vi "PH_TKTDS-30xx.Reset.vi"(0 "i ref in":refnum<vi>, 5 "error IO":errorcluster) -> (14 "i ref out":refnum<vi>, 19 "error out":errorcluster)   [LabVIEW 2014, in "PH_TKTDS-30xx.lvlib"]
doc: "If the connection is established, this VO resets the hardware. It queries the errors which are written to own attributes, if the value has changed."
uses:
  PH_TKTDS-30xx.lvlib
  instr.lib/TKDS3032-PHELIX/tktds3032-PHELIX - Driver np.lvlib
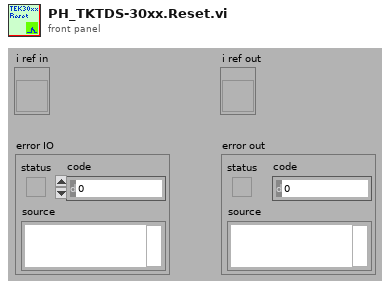
[diagram p1: front panel]
types:
  T1 = typedef "PH_TKTDS-30xx.lvlib/PH_TKTDS-30xx.i attribute.ctl" = cluster{"Default VISA Resource":string, "VISA Resource Name":refnum<visa-resource-name>, "Revision":cluster{"Instrument Driver":string, "Instrument Firmware":string}, "Selftest":cluster{"Result":u32, "Message":string}, "Channels":T2[], "Trigger Configuration":T3, "Acquisition Configuration":T4, "Fetched Waveforms":T5[], "GUI Refs":T6, "GUI Refs Channels":refnum<vi>[], "State":T7, "Error Message":string, "Allow Prdc Loop?":bool}
  T2 = typedef "PH_TKTDS-30xx.lvlib/PH_TKTDS-30xx.Channel Config.ctl" = cluster{"Channel Name":string, "Input Impedance":string, "Max Input Frequency":string, "Vertical Coupling":i32, "Channel Enabled":bool, "Probe Attenuation":dbl, "Vertical Range":dbl, "Vertical Offset":dbl}
  T3 = typedef "PH_TKTDS-30xx.lvlib/PH_TKTDS-30xx.Trigger Config.ctl" = cluster{"Source":string, "Slope":i32, "Level [V]":dbl}
  T4 = typedef "PH_TKTDS-30xx.lvlib/PH_TKTDS-30xx.Acquisition Config.ctl" = cluster{"Time base":dbl, "Record Length":u16, "Start Time":dbl, "Type":i32, "Continuous":bool}
  T5 = typedef "PH_TKTDS-30xx.lvlib/PH_TKTDS-30xx.fetched Waveform.ctl" = cluster{"Source":string, "Actual Points":u32, "Initial X":dbl, "X Increment":dbl, "Waveform Array":dbl[]}
  T6 = typedef "PH_TKTDS-30xx.lvlib/PH_TKTDS-30xx.GUI Refs.ctl" = cluster{"Trigger":refnum<vi>, "Acquisition":refnum<vi>, "Graph":refnum<vi>, "State":refnum<vi>, "Delete":refnum<vi>, "Channel to be positioned":refnum<vi>, "Postion":refnum<vi>, "Display Intensity":refnum<vi>, "VISA Resource":refnum<vi>}
  T7 = typedef "PH_StatusHandler.lvlib/PH_StatusHandler.Status.ctl" = i16
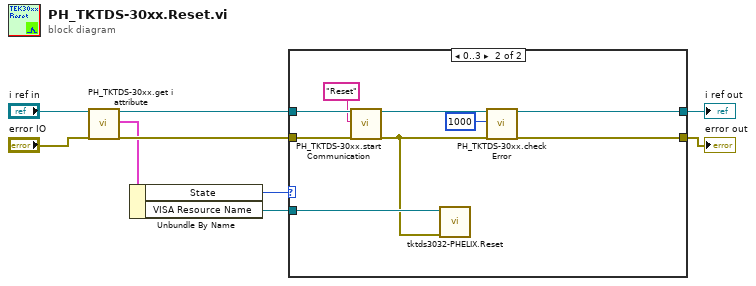
[diagram p0: block diagram]
diagram:
  n1 = call "PH_TKTDS-30xx.get i attribute.vi"("i ref in"="i ref in", "error in (no error)"="error IO") -> ("i ref out"=w2:refnum<vi>, "i attribute"=w4:T1, "error out"=w7:errorcluster)  [unwired: 15 in]
  n2 = Unbundle By Name(w4) -> ("State"=w9:T7, "VISA Resource Name"=w5:refnum<visa-resource-name>)
  n3 = case shown="0..3" w9 {
    tunnel: w2 -> [w11 w20]
    tunnel: w5 -> [_ w19]
    tunnel: [w10 w18] -> w6
    tunnel: w7 -> [w10 w17]
    tunnel: [w11 w16] -> w8
    frame Default {
    }
    frame 0..3 {
      n4 = call "PH_TKTDS-30xx.start Communication.vi"("i ref in"=w20, "Action"="Reset", "error in"=w17) -> ("i ref out"=w15:refnum<vi>, "error out"=w14:errorcluster)  [unwired: 15 in]
      n5 = call "tktds3032-PHELIX.Reset.vi"("error in (no error)"=w14, "VISA Resource Name"=w19) -> ()  [unwired: 8 in, 2 out]
      n6 = call "PH_TKTDS-30xx.check Error.vi"("i ref in"=w15, "Waiting Time [ms]"=u32 1000, "error in"=w14) -> ("i ref out"=w16:refnum<vi>, "error out"=w18:errorcluster)  [unwired: 15 in]
    }
  }
  "i ref out" <- w8
  "error out" <- w6
